vi "Dequeue.vi"(8 "error in (no error)":errorcluster) -> (0 "error out":errorcluster, 1 "Message":string, 3 "Data":variant)   [LabVIEW 2010, in "Template Module.lvlib"]
uses:
  Template Module.lvlib
  Q Ref FGV Command Enum.ctl
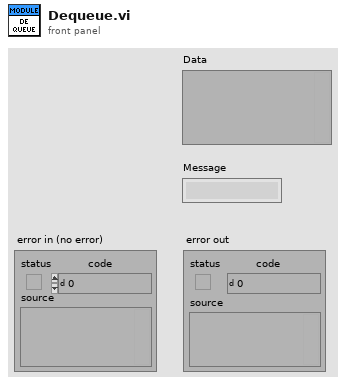
[diagram p1: front panel]
types:
  T1 = typedef "Template Module.lvlib/Q Ref FGV Command Enum.ctl" = enum16{"Create Q", "Get Q", "Flush Q", "Release Q"}
  T2 = typedef "Q Message Cluster.ctl" = cluster{"Message":string, "Data":variant}
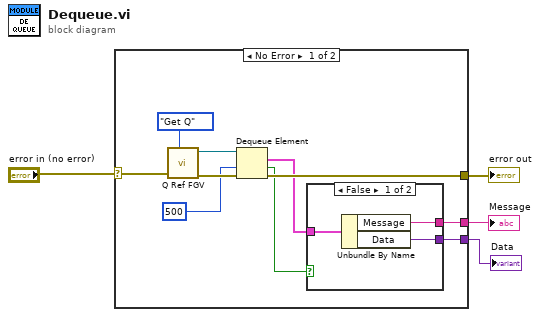
[diagram p0: block diagram]
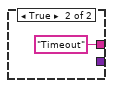
[diagram p2: hidden frame]
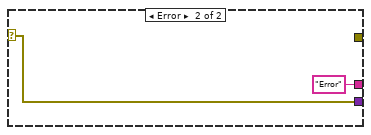
[diagram p3: hidden frame]
diagram:
  n1 = case shown="No Error" "error in (no error)" {
    selector: "error in (no error)" -> [w10 w19]
    tunnel: [w12 _] -> w4
    tunnel: [w6 "Error" ("Message")] -> w2
    tunnel: [w5 w19] -> w1
    frame No Error {
      n2 = call "Q Ref FGV.vi"("Command"=Q_Ref_FGV_Command_Enum."Get Q", "error in (no error)"=w10) -> ("error out"=w11:errorcluster, "Q Ref"=w13:refnum<queue>)  [unwired: 8 in]
      n3 = Dequeue Element(queue=w13, timeout in ms (-1)=500, error in (no error)=w11) -> (element=w7:T2, timed out?=w8:bool, error out=w12:errorcluster)  [unwired: 1 out]
      n4 = case shown="False" w8 {
        tunnel: w7 -> [w17 _]
        tunnel: [w16 "Timeout" ("Message")] -> w6
        tunnel: [w15 _] -> w5
        frame False {
          n5 = Unbundle By Name(w17) -> ("Message"=w16:string, "Data"=w15:variant)
        }
        frame True {
        }
      }
    }
    frame Error {
    }
  }
  "error out" <- w4
  "Message" <- w2
  "Data" <- w1
